vi "EditPageNames UI.vi"(11 "PageNames":string[](array[string])) -> (3 "PageNames out":string[](array[string]))   [LabVIEW 2016]
uses:
  <vilib>/Utility/error.llb/DialogType.ctl
  PanelSplitToolkit/QueueManager.llb/CreatQueue.vi
  PanelSplitToolkit/QueueManager.llb/Insert.vi
  PanelSplitToolkit/QueueManager.llb/Remove.vi
  PanelSplitToolkit/QueueManager.llb/Destroy.vi
panel:
  in  "Card List":i32(listbox)
  in  "Cancel":bool
  in  "OK":bool
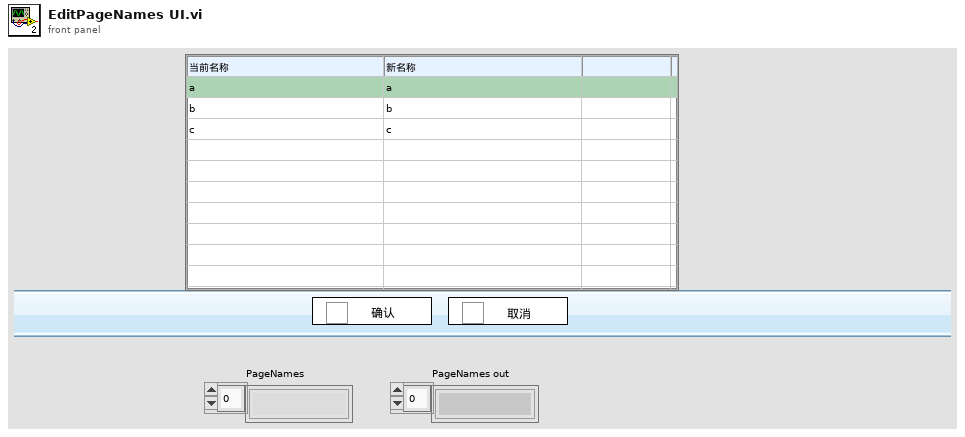
[diagram p1: front panel]
types:
  T1 = cluster{"error":errorcluster, "LocalQ":cluster{"LQName":string, "LQEvent":string, "LQData":variant}, "HighQ":cluster{"HQName":string, "HQEvent":string, "HQData":variant}, "PageNames":string[]}
  T2 = typedef "LVPoint32TypeDef.ctl" = cluster{"Horizontal":i32, "Vertical":i32}
  T3 = typedef "DialogType.ctl" = u16
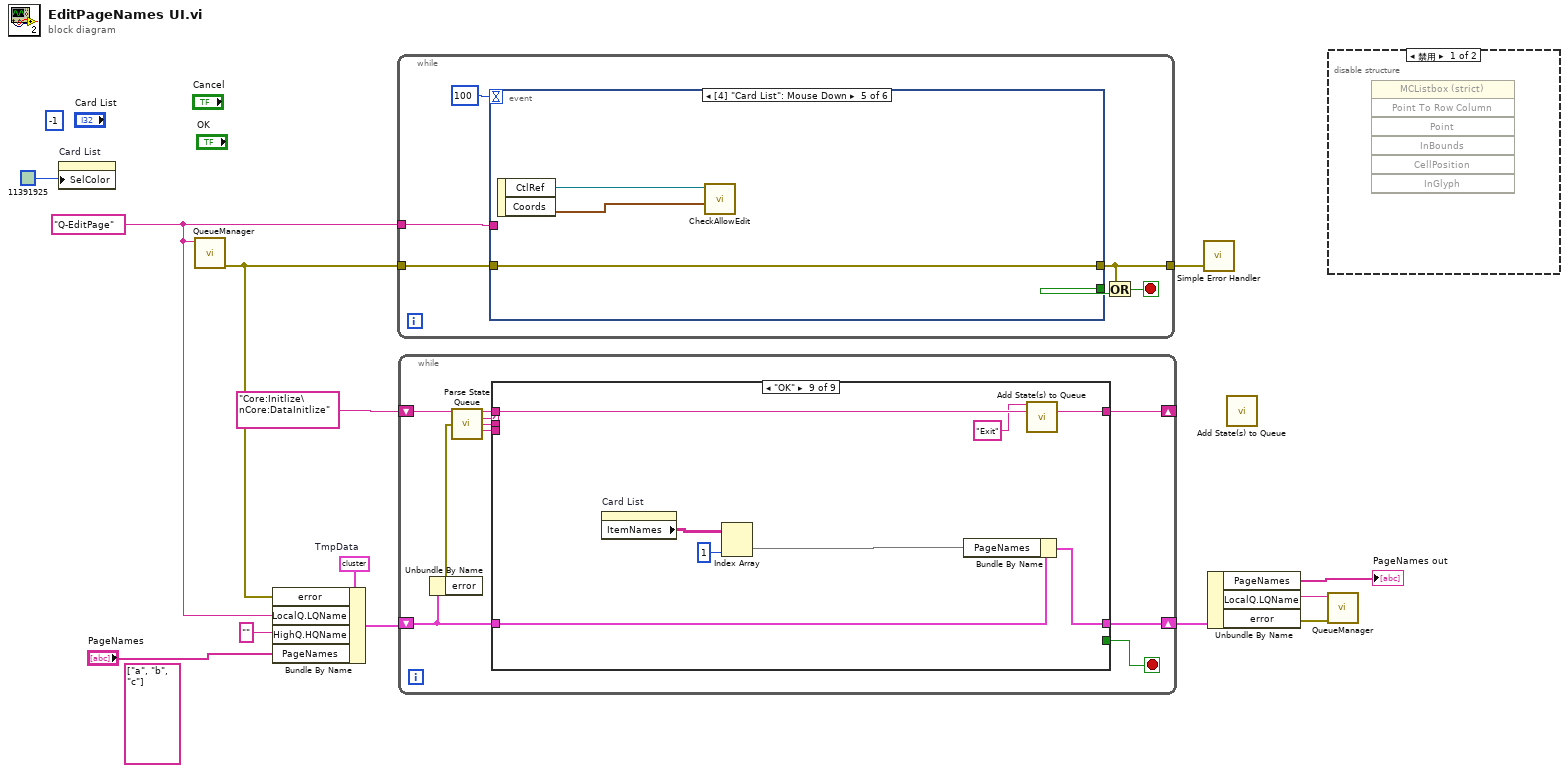
[diagram p0: block diagram]
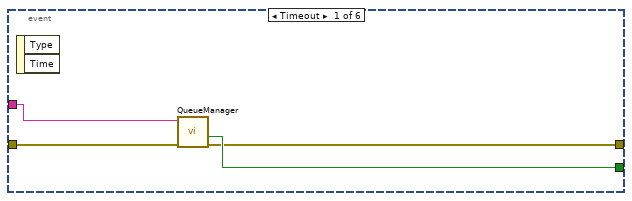
[diagram p3: hidden frame]
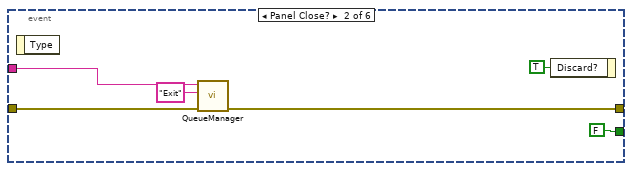
[diagram p4: hidden frame]
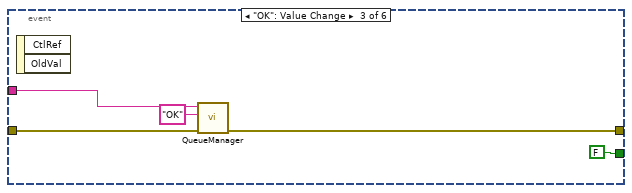
[diagram p5: hidden frame]
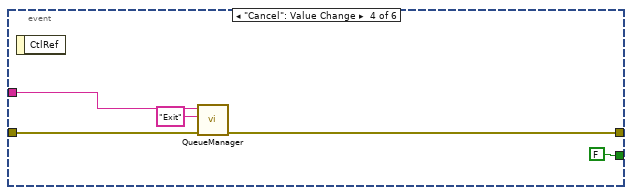
[diagram p6: hidden frame]
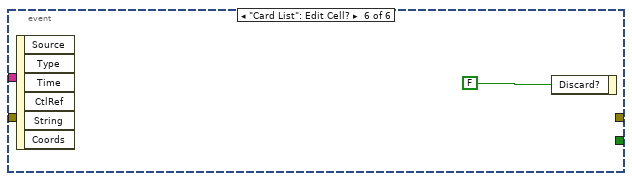
[diagram p7: hidden frame]
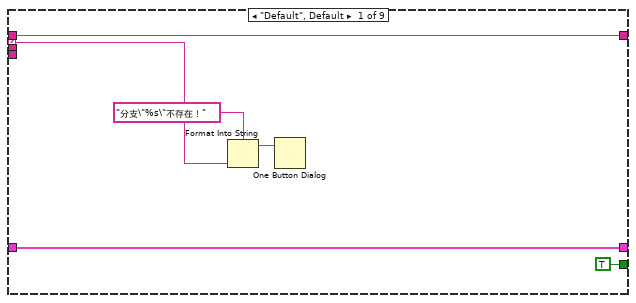
[diagram p8: hidden frame]
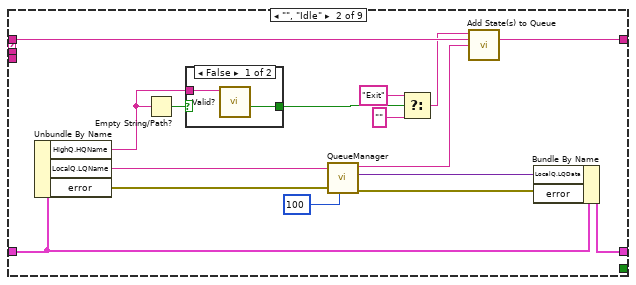
[diagram p9: hidden frame]
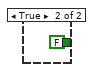
[diagram p10: hidden frame]
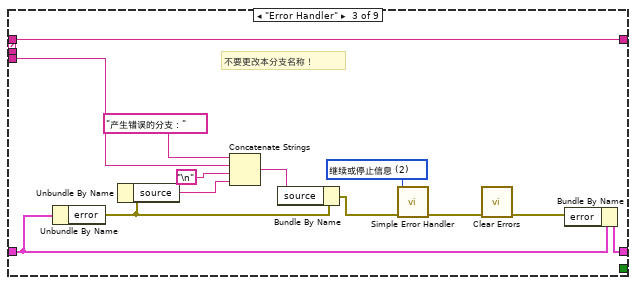
[diagram p11: hidden frame]
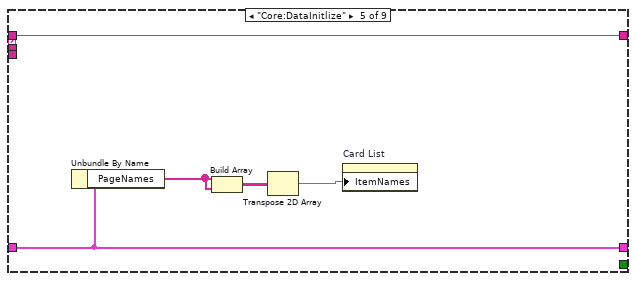
[diagram p13: hidden frame]
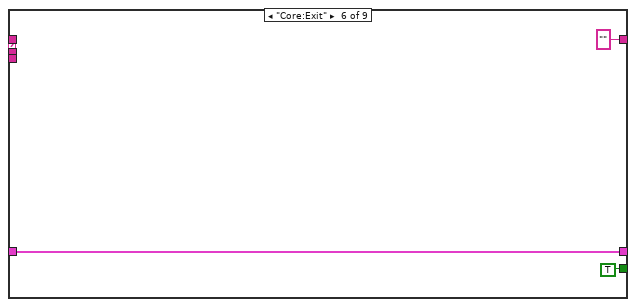
[diagram p14: hidden frame]
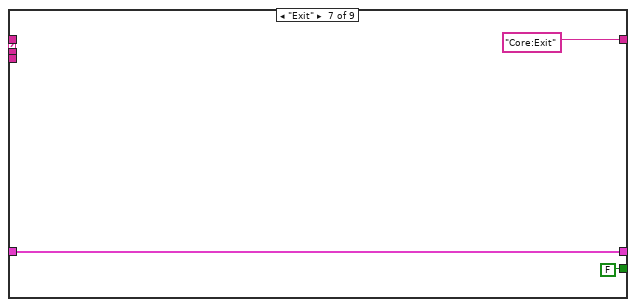
[diagram p15: hidden frame]
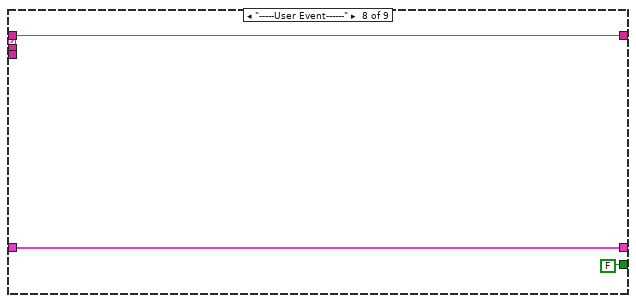
[diagram p16: hidden frame]
diagram:
  (unwired) string[] ["a", "b", "c"] ("PageNames")
  w7 = "Q-EditPage" ("QueueName")
  w9 = T1 {"error"={"status"=FALSE, "code"=0, "source"=""}, "LocalQ"={"LQName"="", "LQEvent"="", "LQData"=variant}, "HighQ"={"HQName"="", "HQEvent"="", "HQData"=variant}, "PageNames"=[]}  # TmpData
  (unwired) -1 ("Card List")
  n1 = property on="Card List" class="MCListbox (strict)"("SelColor"=u32 11391925) -> ()  [unwired: 2 in, 2 out]
  n2 = call-poly "QueueManager.vi"("QueueName"=w7) -> ("error out"=w5:errorcluster)  [unwired: 9 in, 1 out]
  n3 = Bundle By Name(cluster=w9, "error"=w5, "LocalQ.LQName"=w7, "HighQ.HQName"="" ("Caller"), "PageNames"="PageNames") -> (w8:T1)
  n4 = while {
    tunnel: w5 -> [w18]
    tunnel: w7 -> [w19]
    tunnel: [w15] -> w10
    stop <- w16 stop-if-true
    n5 = event shown="[4] \"Card List\": Mouse Down" {
      selector: _ -> [_ _ _ _ _ _]
      dyn-events: _ -> [_ _ _ _ _ _]
      timeout: 100 -> [_ _ _ _ _ _]
      tunnel: [w21 FALSE FALSE FALSE _ _] -> w17
      tunnel: w19 -> [w23 w28 w33 w38 _ _]
      tunnel: w18 -> [w22 w27 w32 w37 w40 _]
      tunnel: [w20 w26 w31 w36 w40 _] -> w15
      event Timeout {
        n6 = event-data() -> ()  [unwired: 1 in, 2 out]
        n7 = call-poly "QueueManager.vi"("error in (no error)"=w22, "Queue Name(unamed)"=w23) -> ("error out"=w20:errorcluster, "Not Exist?"=w21:bool)  [unwired: 8 in]
      }
      event Panel Close? {
        n8 = event-data() -> ()  [unwired: 1 in, 1 out]
        n9 = call-poly "QueueManager.vi"("error in"=w27, "Event"="Exit", "QueueName"=w28) -> ("error out"=w26:errorcluster)  [unwired: 7 in, 1 out]
        n10 = event-data("Discard?"=TRUE ("放弃？")) -> ()  [unwired: 1 in, 1 out]
      }
      event "OK": Value Change {
        n11 = event-data() -> ()  [unwired: 1 in, 2 out]
        n12 = call-poly "QueueManager.vi"("error in"=w32, "Event"="OK", "QueueName"=w33) -> ("error out"=w31:errorcluster)  [unwired: 7 in, 1 out]
      }
      event "Cancel": Value Change {
        n13 = event-data() -> ()  [unwired: 1 in, 1 out]
        n14 = call-poly "QueueManager.vi"("error in"=w37, "Event"="Exit", "QueueName"=w38) -> ("error out"=w36:errorcluster)  [unwired: 7 in, 1 out]
      }
      event "Card List": Mouse Down {
        n15 = event-data() -> ("CtlRef"=w42:refnum<vi>, "Coords"=w41:T2)  [unwired: 1 in]
        n16 = call "CheckAllowEdit.vi"("点"=w41, "ref in"=w42) -> ()  [unwired: 10 in]
      }
      event "Card List": Edit Cell? {
        n17 = event-data() -> ()  [unwired: 1 in, 6 out]
        n18 = event-data("Discard?"=FALSE ("放弃？")) -> ()  [unwired: 1 in, 1 out]
      }
    }
    n19 = Or(x=w15, y=w17) -> (x .or. y?=w16:bool)
  }
  n20 = while {
    shift-right: [w47] -> w11
    shift-left: w8 -> [w48]
    shift-right: [w46] -> _
    shift-left: "Core:Initlize\nCore:DataInitlize" -> [w53]
    stop <- w50 stop-if-true
    n21 = Unbundle By Name(w48) -> ("error"=w49:errorcluster)
    n22 = call "Parse State Queue.vi"("State Queue"=w53, "Error In (no error)"=w49) -> ("Remaining States"=w52:string, "Current State"=w51:string, "Arguments"=w45:string, "PreState"=w44:string)  [unwired: 10 in]
    n23 = case shown="\"OK\"" w51 {
      selector: w51 -> [w57 _ _ _ _ _ _ _ _]
      tunnel: w52 -> [w58 w72 w91 w93 w98 _ _ w105 w110]
      tunnel: w45 -> [_ _ _ _ _ _ _ _ _]
      tunnel: [TRUE _ _ _ _ TRUE FALSE FALSE _] -> w50
      tunnel: w48 -> [w59 w69 w88 w92 w97 w100 w103 w106 w113]
      tunnel: [w59 w74 w87 w92 w97 w100 w103 w106 w111] -> w47
      tunnel: [w58 w71 w91 w93 w98 "" ("Remaining States") "Core:Exit" ("Remaining States") w105 w109] -> w46
      tunnel: w44 -> [_ _ w85 _ _ _ _ _ _]
      frame "Default", Default {
        n24 = Format Into String(format string="分支\"%s\"不存在！" ("格式字符串"), w57) -> (resulting string=w56:string)  [unwired: 2 in, 1 out]
        n25 = One Button Dialog(message=w56) -> ()  [unwired: 1 in, 1 out]
      }
      frame "", "Idle" {
        n26 = Unbundle By Name(w69) -> ("HighQ.HQName"=w63:string, "LocalQ.LQName"=w68:string, "error"=w67:errorcluster)
        n27 = Empty String/Path?(string/path=w63) -> (empty?=w66:bool)
        n28 = case shown="False" w66 {
          tunnel: [w77 FALSE ("Not Exist?")] -> w65
          tunnel: w63 -> [w76 _]
          frame False {
            n29 = call "Valid?.vi"("Queue Name(unamed)"=w76) -> ("Not Exist?"=w77:bool)  [unwired: 9 in, 1 out]
          }
          frame True {
          }
        }
        n30 = call-poly "QueueManager.vi"("Time out(-1)"=100, "error in (no error)"=w67, "Queue Name"=w68) -> ("error out"=w75:errorcluster, "Data"=w73:variant, "Event"=w62:string)  [unwired: 5 in, 1 out]
        n31 = Select(t="Exit" ("Event"), s=w65, f="") -> (s? t:f=w60:string)
        n32 = call "Add State(s) to Queue.vi"("State(s) in Front (\"\")"=w60, "State(s) in (\"\")"=w72, "State(s) at Back (\"\")"=w62) -> ("States Out"=w71:string)  [unwired: 12 in]
        n33 = Bundle By Name(cluster=w69, "LocalQ.LQData"=w73, "error"=w75) -> (w74:T1)
      }
      frame "Error Handler" {
        w86 = T3 2 items=["无对话框", "确定信息", "继续或停止信息", "确定信息＋警告", "继续/停止+警告"] ("type of dialog (OK msg:1)")
        # "不要更改本分支名称！"
        n34 = Unbundle By Name(w88) -> ("error"=w80:errorcluster)
        n35 = Unbundle By Name(w80) -> ("source"=w83:string)
        n36 = Concatenate Strings("产生错误的分支：" ("字符串"), w85, "\n", w83) -> (w81:string)
        n37 = Bundle By Name(cluster=w80, "source"=w81) -> (w79:errorcluster)
        n38 = call <vilib>:"Simple Error Handler.vi"("type of dialog (OK msg:1)"=w86, "error in (no error)"=w79) -> ("error out"=w89:errorcluster)  [unwired: 3 in, 4 out]
        n39 = call <vilib>:"Clear Errors.vi"("error in (no error)"=w89) -> ("error out"=w90:errorcluster)  [unwired: 5 in, 1 out]
        n40 = Bundle By Name(cluster=w88, "error"=w90) -> (w87:T1)
      }
      frame "Core:Initlize" {
      }
      frame "Core:DataInitlize" {
        n41 = Unbundle By Name(w97) -> ("PageNames"=w96:string[])
        n42 = Build Array(w96, w96) -> (w95:string[][])
        n43 = Transpose 2D Array(2D array=w95) -> (transposed array=w94:string[][])
        n44 = property on="Card List" class="MCListbox (strict)"("ItemNames"=w94) -> ()  [unwired: 2 in, 2 out]
      }
      frame "Core:Exit" {
      }
      frame "Exit" {
      }
      frame "-----User Event------" {
      }
      frame "OK" {
        n45 = property on="Card List" class="MCListbox (strict)"() -> ("ItemNames"=w115:string[][])  [unwired: 2 in, 2 out]
        n46 = Index Array(array=w115, index (col)=1 ("禁用的索引 (列)")) -> (element=w112:string[])  [unwired: 1 in]
        n47 = Bundle By Name(cluster=w113, "PageNames"=w112) -> (w111:T1)
        n48 = call "Add State(s) to Queue.vi"("State(s) in Front (\"\")"="Exit" ("State(s) in Front (\"\")"), "State(s) in (\"\")"=w110) -> ("States Out"=w109:string)  [unwired: 13 in]
      }
    }
  }
  n49 = call <vilib>:"Simple Error Handler.vi"("error in (no error)"=w10) -> ()  [unwired: 4 in, 5 out]
  n50 = Unbundle By Name(w11) -> ("PageNames"=→"PageNames out":string[], "LocalQ.LQName"=w6:string, "error"=w12:errorcluster)
  n51 = call "Add State(s) to Queue.vi"() -> ()  [unwired: 15 in, 1 out]
  n52 = call-poly "QueueManager.vi"("error in (no error)"=w12, "QueeuName"=w6) -> ()  [unwired: 9 in, 1 out]
  n53 = disable-structure shown="禁用" {
    frame Disabled {
      n54 = invoke class="MCListbox (strict)" method="Point To Row Column"() -> ()  [unwired: 7 in, 7 out]
    }
    frame Enabled {
    }
  }
